vi "Write bitfile path.vi"(8 "error in":errorcluster, 10 "bitfile path":path, 11 "Targets in":refnum<class "Targets.lvclass">) -> (0 "error out":errorcluster, 3 "Targets out":refnum<class "Targets.lvclass">)   [LabVIEW 2013, in "Targets.lvclass"]
uses:
  Targets.lvclass
  Targets.lvclass/Targets.ctl
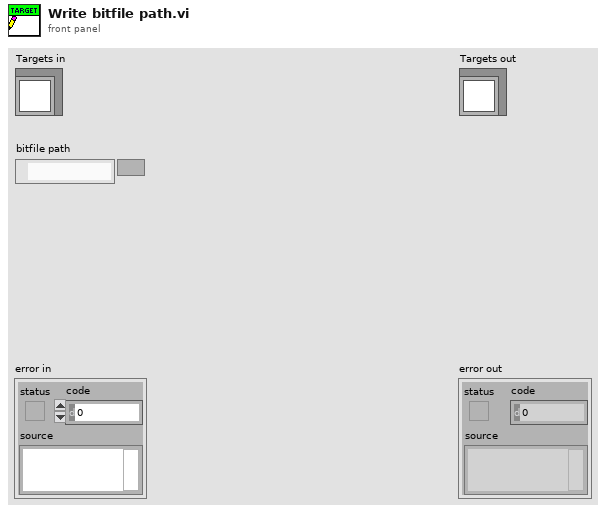
[diagram p1: front panel]
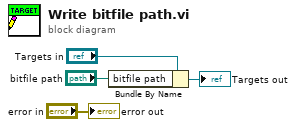
[diagram p0: block diagram]
diagram:
  n1 = Bundle By Name(cluster="Targets in", "bitfile path"="bitfile path") -> (→"Targets out":refnum<class "Targets.lvclass">)
  "error out" <- "error in"
